vi "Build Thermal Chamber TAPI Status Message.vi"(6 "Response Time":string, 7 "Module ID":i32, 8 "error in":errorcluster, 9 "Reply Data":variant, 10 "Request/Broadcast Data":variant, 11 "CtlRef":refnum<vi>) -> (0 "error out":errorcluster, 3 "Message":string)   [LabVIEW 2024, in "Thermal Chamber.lvlib"]
doc: "<b>Note:</b> This VI was modified by the <b>Validate DQMH Module</b> tool to be shared clone reentrant."
uses:
  Thermal Chamber.lvlib
  Class Libraries/Process Controller/Controls/Temp Data--Cluster.ctl
  Class Libraries/Process Controller/Controls/Temperature Units--Enum.ctl
  Class Libraries/Process Controller/Controls/Temp Ramp Rate Data--Cluster.ctl
  Class Libraries/Process Controller/Controls/Rate Units--Enum.ctl
  Class Libraries/Process Controller/_Thermal Process Controller.lvclass
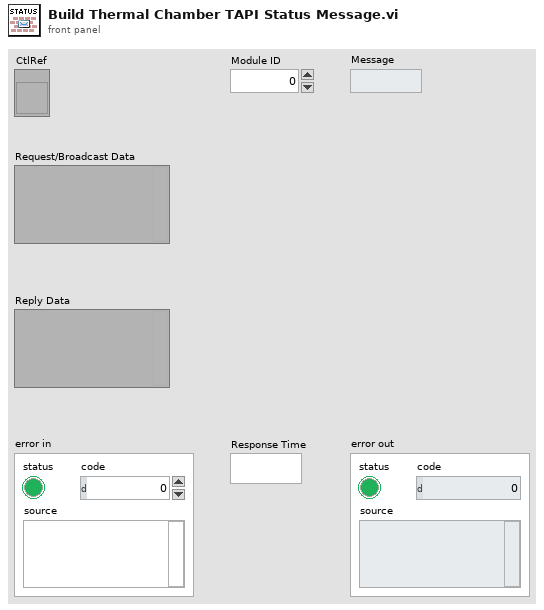
[diagram p1: front panel]
types:
  T1 = typedef "_Thermal Process Controller.lvclass/Temp Data--Cluster.ctl" = cluster{"Temp":dbl, "Temp Units":T2}
  T2 = typedef "_Thermal Process Controller.lvclass/Temperature Units--Enum.ctl" = enum16{"Degrees F", "Degrees C", "Degrees K"}
  T3 = typedef "_Thermal Process Controller.lvclass/Temp Ramp Rate Data--Cluster.ctl" = cluster{"Temp Ramp Rate":dbl, "Temp Units":T2, "Rate Units":T4}
  T4 = typedef "_Thermal Process Controller.lvclass/Rate Units--Enum.ctl" = enum16{"Degrees/Minutes", "Degrees/Hours"}
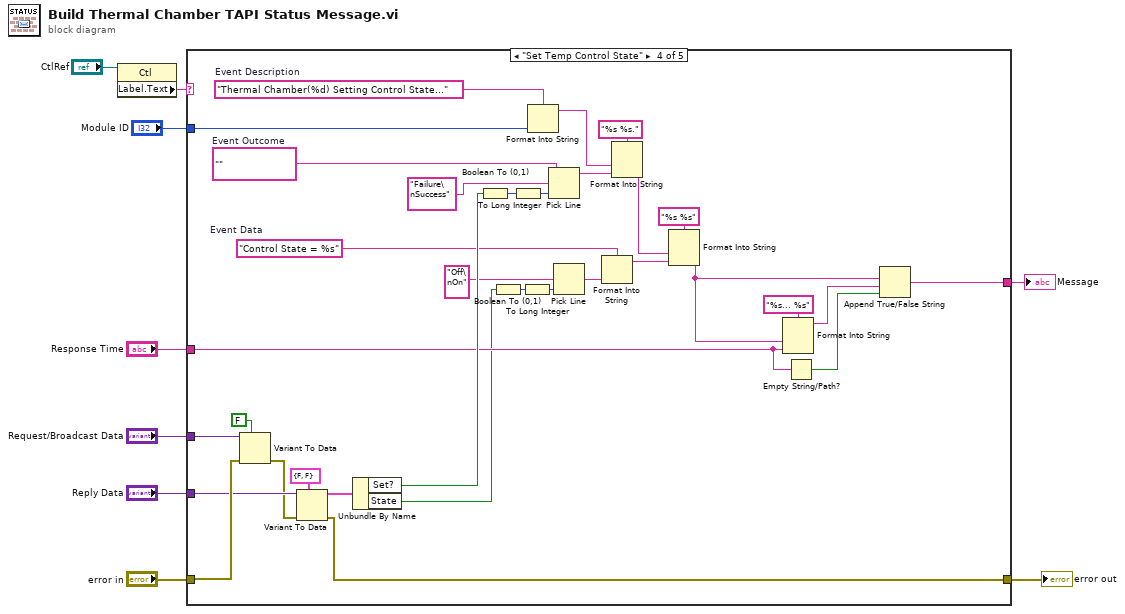
[diagram p0: block diagram]
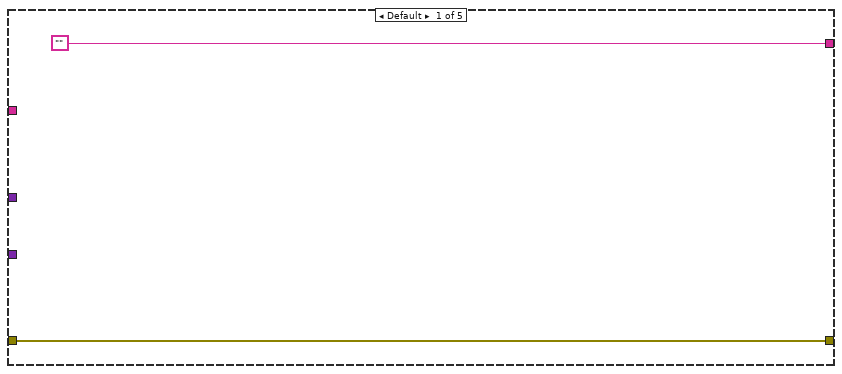
[diagram p2: hidden frame]
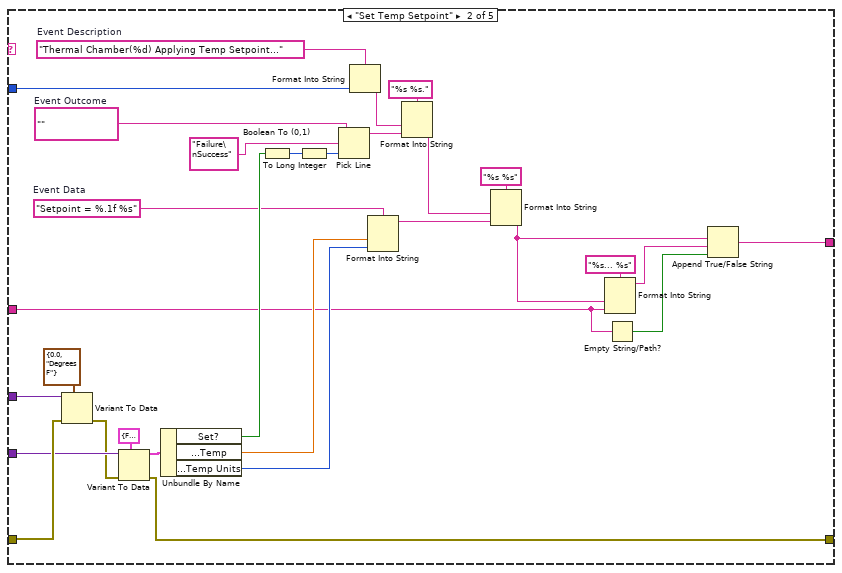
[diagram p3: hidden frame]
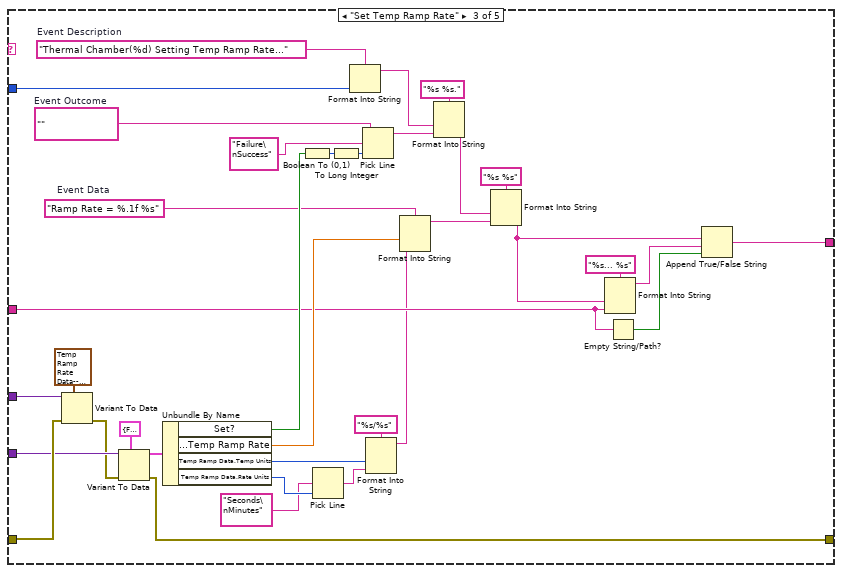
[diagram p4: hidden frame]
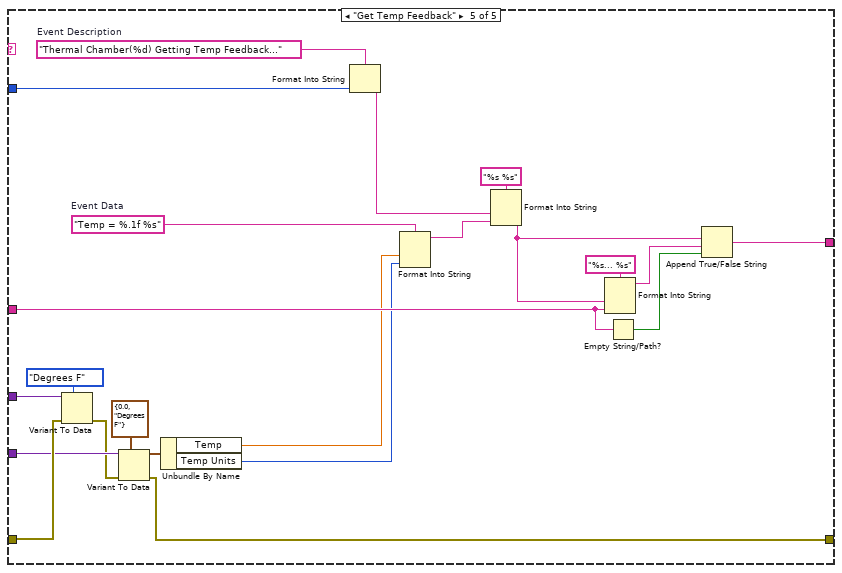
[diagram p5: hidden frame]
diagram:
  n1 = property class="Ctl"(reference="CtlRef") -> ("Label.Text"=w1:string)  [unwired: 1 in, 2 out]
  n2 = case shown="\"Set Temp Control State\"" w1 {
    tunnel: "error in" -> [w10 w35 w71 w104 w128]
    tunnel: [w10 w18 w56 w90 w121] -> w8
    tunnel: "Module ID" -> [_ w40 w75 w108 w130]
    tunnel: "Request/Broadcast Data" -> [_ w37 w72 w105 w129]
    tunnel: "Reply Data" -> [_ w34 w70 w103 w127]
    tunnel: "Response Time" -> [_ w17 w50 w87 w118]
    tunnel: ["" w13 w48 w85 w116] -> w3
    frame Default {
    }
    frame "Set Temp Setpoint" {
      w23 = "Setpoint = %.1f %s"  # Event Data
      w30 = ""  # Event Outcome
      w41 = "Thermal Chamber(%d) Applying Temp Setpoint..."  # Event Description
      n3 = Variant To Data(error in=w35, type=T1 {"Temp"=0.0, "Temp Units"=enum."Degrees F"} ("Temp Setpoint Data"), Variant=w37) -> (error out=w32:errorcluster)  [unwired: 1 out]
      n4 = Variant To Data(error in=w32, type=cluster{"Set?":bool, "Temp Setpoint Data":T1} {"Set?"=FALSE, "Temp Setpoint Data"={"Temp"=0.0, "Temp Units"=enum."Degrees F"}} ("output cluster"), Variant=w34) -> (data=w31:cluster{"Set?":bool, "Temp Setpoint Data":T1}, error out=w18:errorcluster)
      n5 = Unbundle By Name(w31) -> ("Set?"=w26:bool, "Temp Setpoint Data.Temp"=w22:dbl, "Temp Setpoint Data.Temp Units"=w21:T2)
      n6 = Boolean To (0,1)(Boolean=w26) -> (0, 1=w27:i16)
      n7 = To Long Integer(number=w27) -> (32bit integer=w12:i32)
      n8 = Pick Line(string ("")=w30, multi-line string="Failure\nSuccess", line index=w12) -> (output string=w29:string)
      n9 = Format Into String(format string=w41, w40) -> (resulting string=w38:string)  [unwired: 2 in, 1 out]
      n10 = Format Into String(format string=w23, w22, w21) -> (resulting string=w20:string)  [unwired: 2 in, 1 out]
      n11 = Format Into String(format string="%s %s.", w38, w29) -> (resulting string=w19:string)  [unwired: 2 in, 1 out]
      n12 = Format Into String(format string="%s %s", w19, w20) -> (resulting string=w15:string)  [unwired: 2 in, 1 out]
      n13 = Format Into String(format string="%s... %s", w15, w17) -> (resulting string=w14:string)  [unwired: 2 in, 1 out]
      n14 = Empty String/Path?(string/path=w17) -> (empty?=w16:bool)
      n15 = Append True/False String(1:w16, 2:w14, 3:w15) -> (0:w13:string)  [unwired: 1 in]
    }
    frame "Set Temp Ramp Rate" {
      w60 = "Ramp Rate = %.1f %s"  # Event Data
      w67 = ""  # Event Outcome
      w76 = "Thermal Chamber(%d) Setting Temp Ramp Rate..."  # Event Description
      n16 = Variant To Data(error in=w71, type=T3 {"Temp Ramp Rate"=5.0, "Temp Units"=enum."Degrees F", "Rate Units"=enum."Degrees/Minutes"} ("Temp Ramp Data"), Variant=w72) -> (error out=w69:errorcluster)  [unwired: 1 out]
      n17 = Variant To Data(error in=w69, type=cluster{"Set?":bool, "Temp Ramp Data":T3} {"Set?"=FALSE, "Temp Ramp Data"={"Temp Ramp Rate"=0.0, "Temp Units"=enum."Degrees F", "Rate Units"=enum."Degrees/Minutes"}} ("output cluster"), Variant=w70) -> (data=w68:cluster{"Set?":bool, "Temp Ramp Data":T3}, error out=w56:errorcluster)
      n18 = Unbundle By Name(w68) -> ("Set?"=w63:bool, "Temp Ramp Data.Temp Ramp Rate"=w59:dbl, "Temp Ramp Data.Temp Units"=w55:T2, "Temp Ramp Data.Rate Units"=w47:T4)
      n19 = Boolean To (0,1)(Boolean=w63) -> (0, 1=w64:i16)
      n20 = Pick Line(multi-line string="Seconds\nMinutes", line index=w47) -> (output string=w53:string)  [unwired: 1 in]
      n21 = To Long Integer(number=w64) -> (32bit integer=w42:i32)
      n22 = Format Into String(format string=w76, w75) -> (resulting string=w73:string)  [unwired: 2 in, 1 out]
      n23 = Pick Line(string ("")=w67, multi-line string="Failure\nSuccess", line index=w42) -> (output string=w66:string)
      n24 = Format Into String(format string="%s/%s", w55, w53) -> (resulting string=w45:string)  [unwired: 2 in, 1 out]
      n25 = Format Into String(format string=w60, w59, w45) -> (resulting string=w58:string)  [unwired: 2 in, 1 out]
      n26 = Format Into String(format string="%s %s.", w73, w66) -> (resulting string=w57:string)  [unwired: 2 in, 1 out]
      n27 = Format Into String(format string="%s %s", w57, w58) -> (resulting string=w52:string)  [unwired: 2 in, 1 out]
      n28 = Format Into String(format string="%s... %s", w52, w50) -> (resulting string=w51:string)  [unwired: 2 in, 1 out]
      n29 = Empty String/Path?(string/path=w50) -> (empty?=w49:bool)
      n30 = Append True/False String(1:w49, 2:w51, 3:w52) -> (0:w48:string)  [unwired: 1 in]
    }
    frame "Set Temp Control State" {
      w93 = "Control State = %s"  # Event Data
      w100 = ""  # Event Outcome
      w109 = "Thermal Chamber(%d) Setting Control State..."  # Event Description
      n31 = Variant To Data(error in=w104, type=FALSE, Variant=w105) -> (error out=w102:errorcluster)  [unwired: 1 out]
      n32 = Variant To Data(error in=w102, type=cluster{"Set?":bool, "State":bool} {"Set?"=FALSE, "State"=FALSE} ("cluster"), Variant=w103) -> (data=w101:cluster{"Set?":bool, "State":bool}, error out=w90:errorcluster)
      n33 = Unbundle By Name(w101) -> ("Set?"=w96:bool, "State"=w80:bool)
      n34 = Boolean To (0,1)(Boolean=w96) -> (0, 1=w97:i16)
      n35 = Boolean To (0,1)(Boolean=w80) -> (0, 1=w82:i16)
      n36 = To Long Integer(number=w97) -> (32bit integer=w77:i32)
      n37 = To Long Integer(number=w82) -> (32bit integer=w78:i32)
      n38 = Format Into String(format string=w109, w108) -> (resulting string=w106:string)  [unwired: 2 in, 1 out]
      n39 = Pick Line(string ("")=w100, multi-line string="Failure\nSuccess", line index=w77) -> (output string=w99:string)
      n40 = Pick Line(multi-line string="Off\nOn", line index=w78) -> (output string=w79:string)  [unwired: 1 in]
      n41 = Format Into String(format string=w93, w79) -> (resulting string=w92:string)  [unwired: 2 in, 1 out]
      n42 = Format Into String(format string="%s %s.", w106, w99) -> (resulting string=w91:string)  [unwired: 2 in, 1 out]
      n43 = Format Into String(format string="%s %s", w91, w92) -> (resulting string=w89:string)  [unwired: 2 in, 1 out]
      n44 = Format Into String(format string="%s... %s", w89, w87) -> (resulting string=w88:string)  [unwired: 2 in, 1 out]
      n45 = Empty String/Path?(string/path=w87) -> (empty?=w86:bool)
      n46 = Append True/False String(1:w86, 2:w88, 3:w89) -> (0:w85:string)  [unwired: 1 in]
    }
    frame "Get Temp Feedback" {
      w123 = "Temp = %.1f %s"  # Event Data
      w131 = "Thermal Chamber(%d) Getting Temp Feedback..."  # Event Description
      n47 = Variant To Data(error in=w128, type=Temperature_Units--Enum."Degrees F" ("Temp Units"), Variant=w129) -> (error out=w126:errorcluster)  [unwired: 1 out]
      n48 = Variant To Data(error in=w126, type=T1 {"Temp"=0.0, "Temp Units"=enum."Degrees F"} ("Temp Feedback Data"), Variant=w127) -> (data=w113:T1, error out=w121:errorcluster)
      n49 = Unbundle By Name(w113) -> ("Temp"=w111:dbl, "Temp Units"=w112:T2)
      n50 = Format Into String(format string=w131, w130) -> (resulting string=w110:string)  [unwired: 2 in, 1 out]
      n51 = Format Into String(format string=w123, w111, w112) -> (resulting string=w122:string)  [unwired: 2 in, 1 out]
      n52 = Format Into String(format string="%s %s", w110, w122) -> (resulting string=w120:string)  [unwired: 2 in, 1 out]
      n53 = Format Into String(format string="%s... %s", w120, w118) -> (resulting string=w119:string)  [unwired: 2 in, 1 out]
      n54 = Empty String/Path?(string/path=w118) -> (empty?=w117:bool)
      n55 = Append True/False String(1:w117, 2:w119, 3:w120) -> (0:w116:string)  [unwired: 1 in]
    }
  }
  "error out" <- w8
  "Message" <- w3
